vi "5900PRStatus.vi"(0 "VISA resource name":refnum<visa-resource-name>="GPIB::1") -> (2 "Panametrics Settings":T1={"ENERGY (uJ)"=0, "DAMPING (Ohm)"=0, "HP FILT (KHz) "=1, "LP FILT (MHz)"=0, "MODE"=0, "PRF (KHz)"=0, "GAIN (db)"=0, "COARSE ATTENUATION"=0, "FINE ATTENUATION"=0} {"FINE ATTENUATION" items=["00.0", "00.5", "01.0", "01.5", "02.0", "02.5", "03.0", "03.5", "04.0", "04.5", "05.0", "05.5", "06.0", "06.5", "07.0", "07.5", "08.0", "08.5", "09.0", "09.5", "10.0", "10.5", "11.0", "11.5", "12.0", "12.5", "13.0", "13.5", "14.0", "14.5", "15.0", "15.5"]; "COARSE ATTENUATION" items=["00.0", "10.0", "20.0", "30.0", "40.0", "50.0"]; "GAIN (db)" items=["26.0", "40.0", "54.0"]; "PRF (KHz)" items=["XREMT", "EXBNC", "0.200", "0.500", "1.000", "2.000", "5.000", "10.00", "20.00"]; "MODE" items=["P/ E", "THRU", "RPP", "EXT_PLSR"]; "LP FILT (MHz)" items=["20", "50", "100", "200"]; "HP FILT (KHz)" items=["1", "1000", "3000", "10000"]; "DAMPING (Ohm)" items=["7", "10", "16", "20", "26", "30", "40", "50"]; "ENERGY (uJ)" items=["1", "2", "4", "8", "16", "32"]}, 3 "Pan Scan Settings":T2, 4 "ATTENUATORS(db)":dbl format="%.2f", 5 "no 5900?":bool)   [LabVIEW 2022 SP3]
uses:
  Pana5900.ctl
panel:
  out "Array":i32[](array[numeric])
  # "This VI returns the present setting of the 5900PR"
  # "(Old form)"
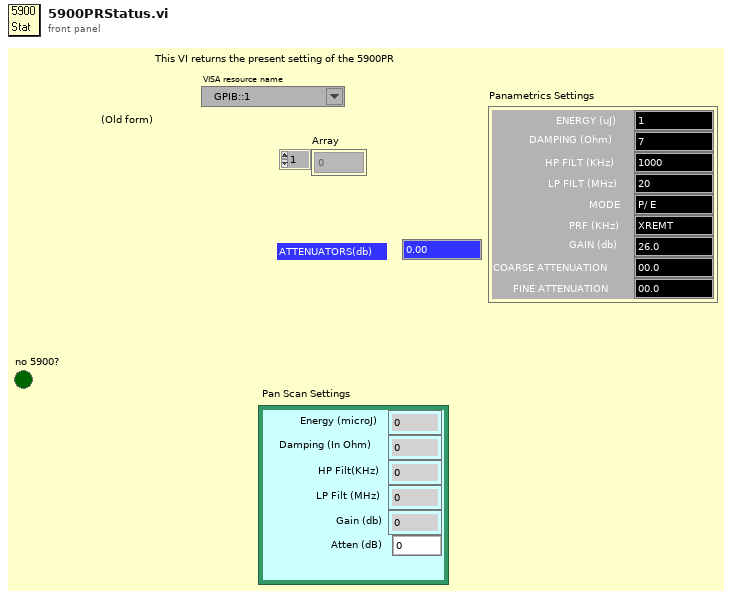
[diagram p1: front panel]
types:
  T1 = typedef "Pana5900.ctl" = cluster{"ENERGY (uJ)":u16, "DAMPING (Ohm)":u16, "HP FILT (KHz) ":u16, "LP FILT (MHz)":u16, "MODE":u16, "PRF (KHz)":u16, "GAIN (db)":u16, "COARSE ATTENUATION":u16, "FINE ATTENUATION":u16}
  T2 = cluster{"Energy (microJ)":u8, "Damping (In Ohm)":u8, "HP Filt(KHz) ":u8, "LP Filt (MHz)":u8, "Gain (db)":u8, "Atten (dB)":sgl}
  T3 = cluster{"[0]":i32, "[1]":i32, "[2]":i32, "[3]":i32, "[4]":i32, "[5]":i32, "[6]":i32, "[7]":i32}
  T4 = cluster{"[5]":i32, "[2]":i32, "[1]":i32, "[0]":i32, "[3]":i32, "[6]":i32}
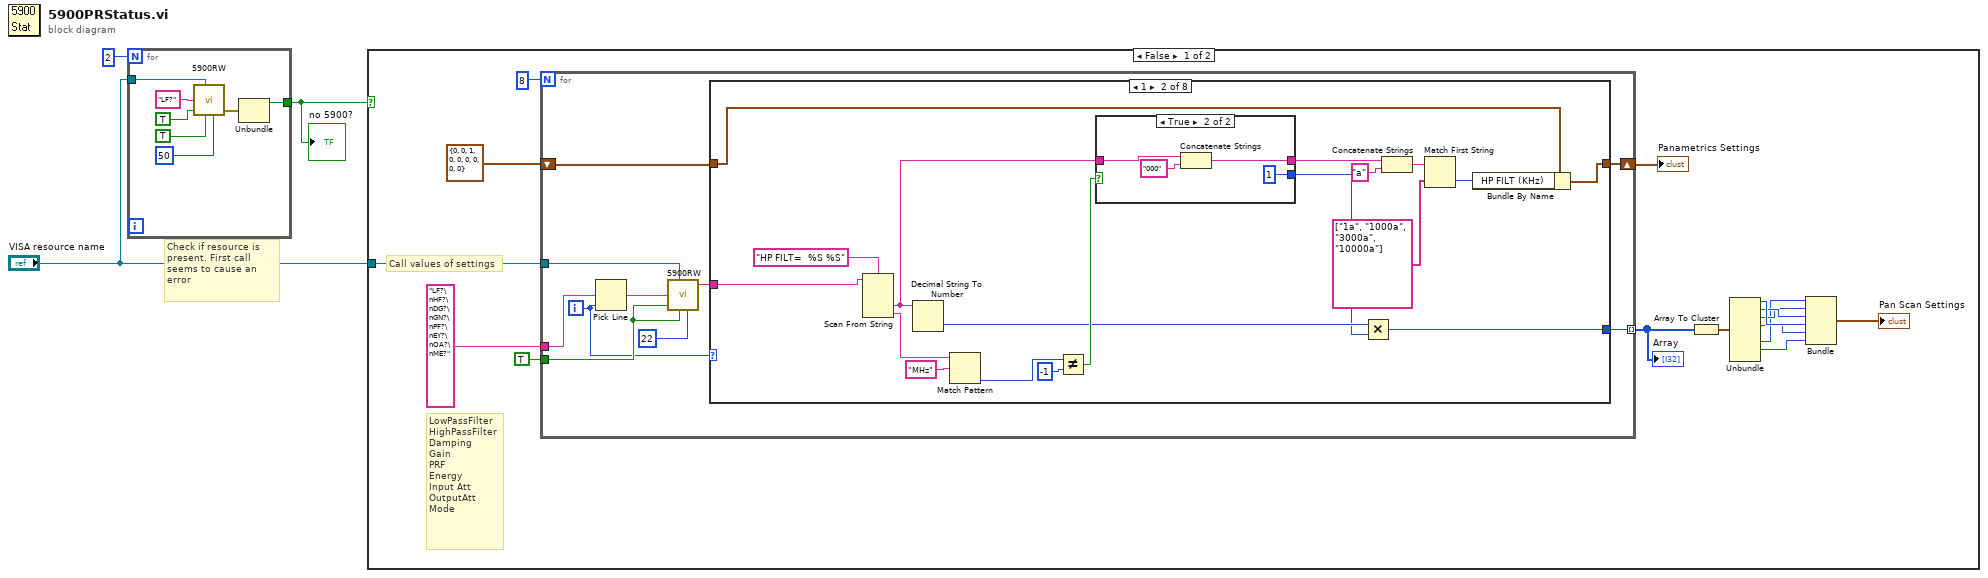
[diagram p0: block diagram]
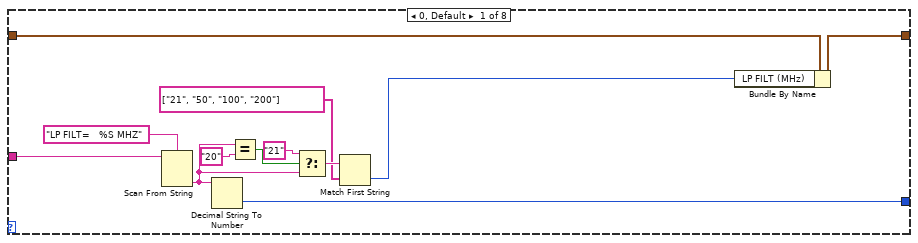
[diagram p2: hidden frame]
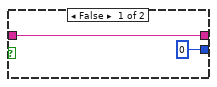
[diagram p3: hidden frame]
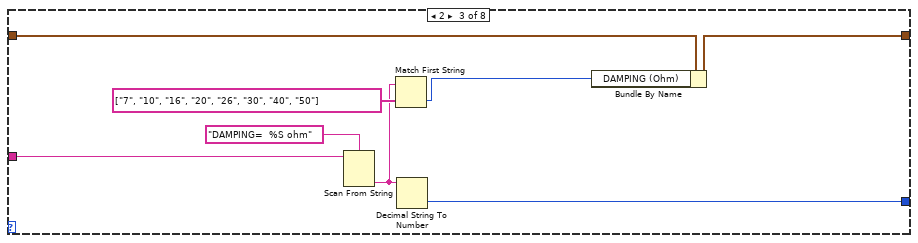
[diagram p4: hidden frame]
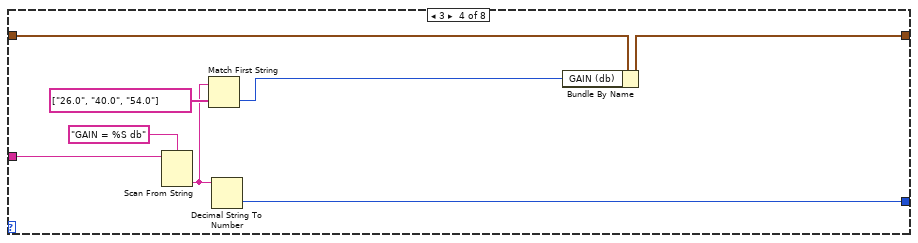
[diagram p5: hidden frame]
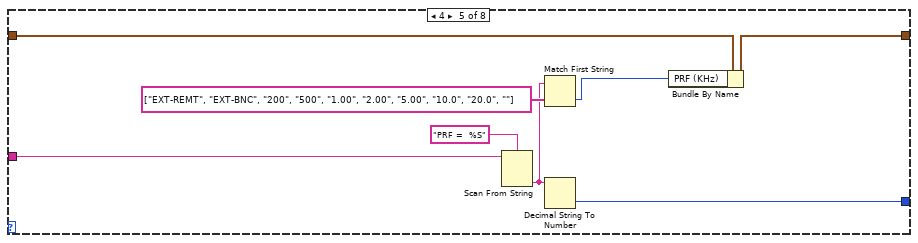
[diagram p6: hidden frame]
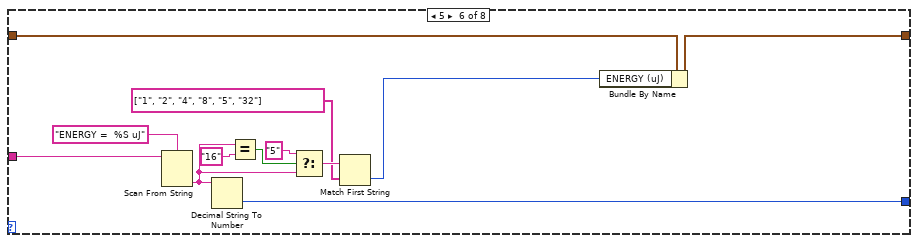
[diagram p7: hidden frame]
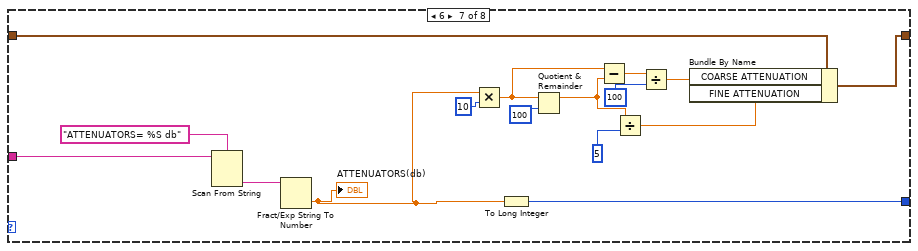
[diagram p8: hidden frame]
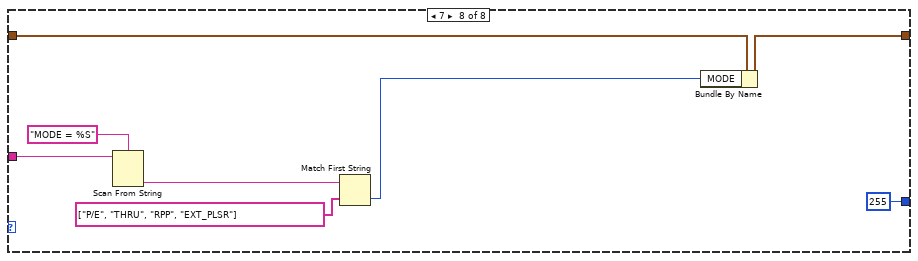
[diagram p9: hidden frame]
diagram:
  # "Check if resource is present. First call seems to cause an error"
  n1 = for {
    N: 2 -> [_]
    tunnel: "VISA resource name" -> [w7]
    tunnel: [w5] -> w2
    n2 = call "5900RW.vi"("VISA resource name"=w7, "ENTER STRING"="LF?", "Read ?"=TRUE, "Write ?"=TRUE, "# bytes\nto read"=50) -> ("error out"=w6:errorcluster)  [unwired: 4 out]
    n3 = Unbundle(w6) -> ("status"=w5:bool)  [unwired: 2 out]
  }
  "no 5900?" <- w2
  n4 = case shown="False" w2 {
    tunnel: "VISA resource name" -> [w23 _]
    frame False {
      # "Call values of settings"
      # "LowPassFilter\nHighPassFilter\nDamping\nGain\nPRF\nEnergy\nInput Att\nOutputAtt\nMode"
      n5 = for {
        N: 8 -> [_]
        tunnel: TRUE -> [w35]
        tunnel: "LF?\nHF?\nDG?\nGN?\nPF?\nEY?\nOA?\nME?" -> [w33]
        tunnel: w23 -> [w30]
        tunnel: [w28] -> w21 mode=indexing
        shift-right: [w27] -> w11
        shift-left: T1 {"ENERGY (uJ)"=0, "DAMPING (Ohm)"=0, "HP FILT (KHz) "=1, "LP FILT (MHz)"=0, "MODE"=0, "PRF (KHz)"=0, "GAIN (db)"=0, "COARSE ATTENUATION"=0, "FINE ATTENUATION"=0} ("Panametrics Settings") -> [w26]
        i -> [w32]
        n6 = Pick Line(multi-line string=w33, line index=w32) -> (output string=w34:string)  [unwired: 1 out]
        n7 = call "5900RW.vi"("VISA resource name"=w30, "ENTER STRING"=w34, "Read ?"=w35, "Write ?"=w35, "# bytes\nto read"=22) -> ("Characters Read"=w31:string)  [unwired: 1 in, 3 out]
        n8 = case shown="1" w32 {
          tunnel: w31 -> [w41 w56 w77 w85 w93 w101 w121 w128]
          tunnel: [w39 w48 w75 w83 w91 w99 w120 255] -> w28
          tunnel: [w37 w49 w73 w81 w89 w97 w112 w125] -> w27
          tunnel: w26 -> [w38 w51 w74 w82 w90 w98 w119 w126]
          frame 0, Default {
            n9 = Scan From String(format string="LP FILT=   %S MHZ", input string=w41) -> (output 1=w40:string)  [unwired: 2 in, 4 out]
            n10 = Decimal String To Number(string=w40) -> (number=w39:i32)  [unwired: 2 in, 1 out]
            n11 = Equal?(x=w40, y="20") -> (x = y?=w44:bool)
            n12 = Select(t="21", s=w44, f=w40) -> (s? t:f=w47:string)
            n13 = Match First String(2:string[] ["21", "50", "100", "200"], 3:w47) -> (0:w36:i32)  [unwired: 1 out]
            n14 = Bundle By Name(cluster=w38, "LP FILT (MHz)"=w36) -> (w37:T1)
          }
          frame 1 {
            n15 = Scan From String(format string="HP FILT=  %S %S", input string=w56) -> (output 1=w54:string, output 2=w55:string)  [unwired: 2 in, 5 out]
            n16 = Decimal String To Number(string=w54) -> (number=w53:i32)  [unwired: 2 in, 1 out]
            n17 = Match Pattern(string=w55, regular expression="MHz") -> (offset past match=w59:i32)  [unwired: 4 out]
            n18 = Not Equal?(x=w59, y=-1) -> (x != y?=w61:bool)
            n19 = case shown="True" w61 {
              tunnel: w54 -> [w67 w69]
              tunnel: [w67 w70] -> w63
              tunnel: [0 1] -> w52
              frame False {
              }
              frame True {
                n20 = Concatenate Strings(w69, "000") -> (w70:string)
              }
            }
            n21 = Multiply(x=w53, y=w52) -> (x*y=w48:i32)
            n22 = Concatenate Strings(w63, "a") -> (w64:string)
            n23 = Match First String(2:string[] ["1a", "1000a", "3000a", "10000a"], 3:w64) -> (0:w50:i32)  [unwired: 1 out]
            n24 = Bundle By Name(cluster=w51, "HP FILT (KHz)"=w50) -> (w49:T1)
          }
          frame 2 {
            n25 = Scan From String(format string="DAMPING=  %S ohm", input string=w77) -> (output 1=w76:string)  [unwired: 2 in, 4 out]
            n26 = Match First String(2:string[] ["7", "10", "16", "20", "26", "30", "40", "50"], 3:w76) -> (0:w72:i32)  [unwired: 1 out]
            n27 = Decimal String To Number(string=w76) -> (number=w75:i32)  [unwired: 2 in, 1 out]
            n28 = Bundle By Name(cluster=w74, "DAMPING (Ohm)"=w72) -> (w73:T1)
          }
          frame 3 {
            n29 = Scan From String(format string="GAIN = %S db", input string=w85) -> (output 1=w84:string)  [unwired: 2 in, 4 out]
            n30 = Match First String(2:string[] ["26.0", "40.0", "54.0"], 3:w84) -> (0:w80:i32)  [unwired: 1 out]
            n31 = Decimal String To Number(string=w84) -> (number=w83:i32)  [unwired: 2 in, 1 out]
            n32 = Bundle By Name(cluster=w82, "GAIN (db)"=w80) -> (w81:T1)
          }
          frame 4 {
            n33 = Scan From String(format string="PRF =  %S", input string=w93) -> (output 1=w92:string)  [unwired: 2 in, 4 out]
            n34 = Match First String(2:string[] ["EXT-REMT", "EXT-BNC", "200", "500", "1.00", "2.00", "5.00", "10.0", "20.0", ""], 3:w92) -> (0:w88:i32)  [unwired: 1 out]
            n35 = Decimal String To Number(string=w92) -> (number=w91:i32)  [unwired: 2 in, 1 out]
            n36 = Bundle By Name(cluster=w90, "PRF (KHz)"=w88) -> (w89:T1)
          }
          frame 5 {
            n37 = Scan From String(format string="ENERGY =  %S uJ", input string=w101) -> (output 1=w100:string)  [unwired: 2 in, 4 out]
            n38 = Decimal String To Number(string=w100) -> (number=w99:i32)  [unwired: 2 in, 1 out]
            n39 = Equal?(x=w100, y="16") -> (x = y?=w104:bool)
            n40 = Select(t="5", s=w104, f=w100) -> (s? t:f=w107:string)
            n41 = Match First String(2:string[] ["1", "2", "4", "8", "5", "32"], 3:w107) -> (0:w96:i32)  [unwired: 1 out]
            n42 = Bundle By Name(cluster=w98, "ENERGY (uJ)"=w96) -> (w97:T1)
          }
          frame 6 {
            n43 = Scan From String(format string="ATTENUATORS= %S db", input string=w121) -> (output 1=w123:string)  [unwired: 2 in, 4 out]
            n44 = Fract/Exp String To Number(string=w123) -> (number=w111:dbl)  [unwired: 4 out]
            "ATTENUATORS(db)" <- w111
            n45 = Multiply(x=w111, y=10) -> (x*y=w117:dbl)
            n46 = To Long Integer(number=w111) -> (32bit integer=w120:i32)
            n47 = Quotient & Remainder(x=w117, y=100) -> (x-y*floor(x/y)=w116:dbl)  [unwired: 1 out]
            n48 = Subtract(x=w117, y=w116) -> (x-y=w110:dbl)
            n49 = Divide(x=w116, y=5) -> (x/y=w109:dbl)
            n50 = Divide(x=w110, y=100) -> (x/y=w108:dbl)
            n51 = Bundle By Name(cluster=w119, "COARSE ATTENUATION"=w108, "FINE ATTENUATION"=w109) -> (w112:T1)
          }
          frame 7 {
            n52 = Scan From String(format string="MODE = %S", input string=w128) -> (output 1=w130:string)  [unwired: 2 in, 4 out]
            n53 = Match First String(2:string[] ["P/E", "THRU", "RPP", "EXT_PLSR"], 3:w130) -> (0:w124:i32)  [unwired: 1 out]
            n54 = Bundle By Name(cluster=w126, "MODE"=w124) -> (w125:T1)
          }
        }
      }
      "Array" <- w21
      "Panametrics Settings" <- w11
      n55 = Array To Cluster(array=w21) -> (cluster=w20:T3)
      n56 = Unbundle(w20) -> ("[0]"=w17:i32, "[1]"=w16:i32, "[2]"=w15:i32, "[3]"=w13:i32, "[5]"=w14:i32, "[6]"=w19:i32)  [unwired: 2 out]
      n57 = Bundle("[5]"=w14, "[2]"=w15, "[1]"=w16, "[0]"=w17, "[3]"=w13, "[6]"=w19) -> (→"Pan Scan Settings":T4)  [unwired: 1 in]
    }
    frame True {
    }
  }
